vi "Variant_to_Fixed_point.vi"(8 "Error in":errorcluster, 11 "Value (in)":variant) -> (0 "Error out":errorcluster, 2 "Value (string)":string, 3 "Value (out)":fxp<+/-,8,8>)   [LabVIEW 2012]
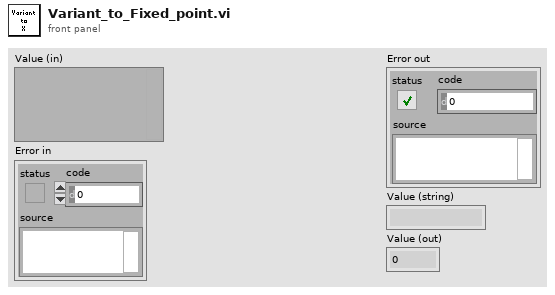
[diagram p1: front panel]
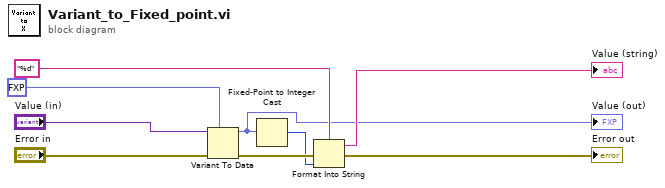
[diagram p0: block diagram]
diagram:
  n1 = Variant To Data(error in="Error in", type=fxp<+/-,32,16> 0.0 ("fixed-point"), Variant="Value (in)") -> (data=w1:fxp<+/-,32,16>, error out=w9:errorcluster)
  "Value (out)" <- w1
  n2 = Fixed-Point to Integer Cast(1:w1) -> (0:w2:i32)
  n3 = Format Into String(format string="%d", error in=w9, w2) -> (resulting string=→"Value (string)":string, error out=→"Error out":errorcluster)  [unwired: 1 in]
